vi "create_process_list (SubVI).vi"(0 "Synth settings:":T1={"start volt (V)"=1.0, "stop volt (V) "=1.0, "# V Steps"=1, "start freq (Hz)"=2000.0, "stop freq (Hz) "=2000.0, "# F steps"=1, "dc offset?"=FALSE, "start DC (V)"=0.5, "stop DC (V)"=0.5, "# DC steps "=1, "Set synth\n(HP33120A)?"=FALSE, "Use arbitrary\nwaveform?"=FALSE, "Arb waveform name:"=""}, 1 "DC supply settings:":T5, 2 "Electrode settings:":T2={"DC volts (V):\n"=[], "Electrode to sweep:"=0, "start volt (V)"=0.0, "stop volt (V) "=0.0, "# V Steps"=1, "start freq (Hz)"=41.0, "stop freq (Hz) "=41.0, "# F steps"=1, "start DC (V)"=0.0, "stop DC (V)"=0.0, "# DC steps "=1, "Digitize electrode\ndrives?"=FALSE, "Sweep electrode?"=FALSE, "Add 0.5*V DC \noffset for amp?"=FALSE, "Use electrode \nconfig file?"=FALSE, "Path"=path ""}, 3 "Stage settings:":T3={"Set stage?"=FALSE, "start X (um)"=0.0, "stop X (um) "=0.0, "# X Steps"=1, "start Y (um)"=0.0, "stop Y (um) "=0.0, "# Y steps"=1, "start Z (um)"=0.0, "stop Z (um)"=0.0, "# Z steps "=1, "Sweep?"=FALSE, "Dir to sweep"=0, "Amplitude (um)"=0.0, "Frequency (Hz)"=41.0} {"Dir to sweep" items=["X", "Y", "Z"]}) -> (6 "Process list":T4(array[cluster]))   [LabVIEW 2014]
panel:
  # "0"
  # "1"
  # "2"
  # "3"
  # "4"
  # "5"
  # "6"
  # "7"
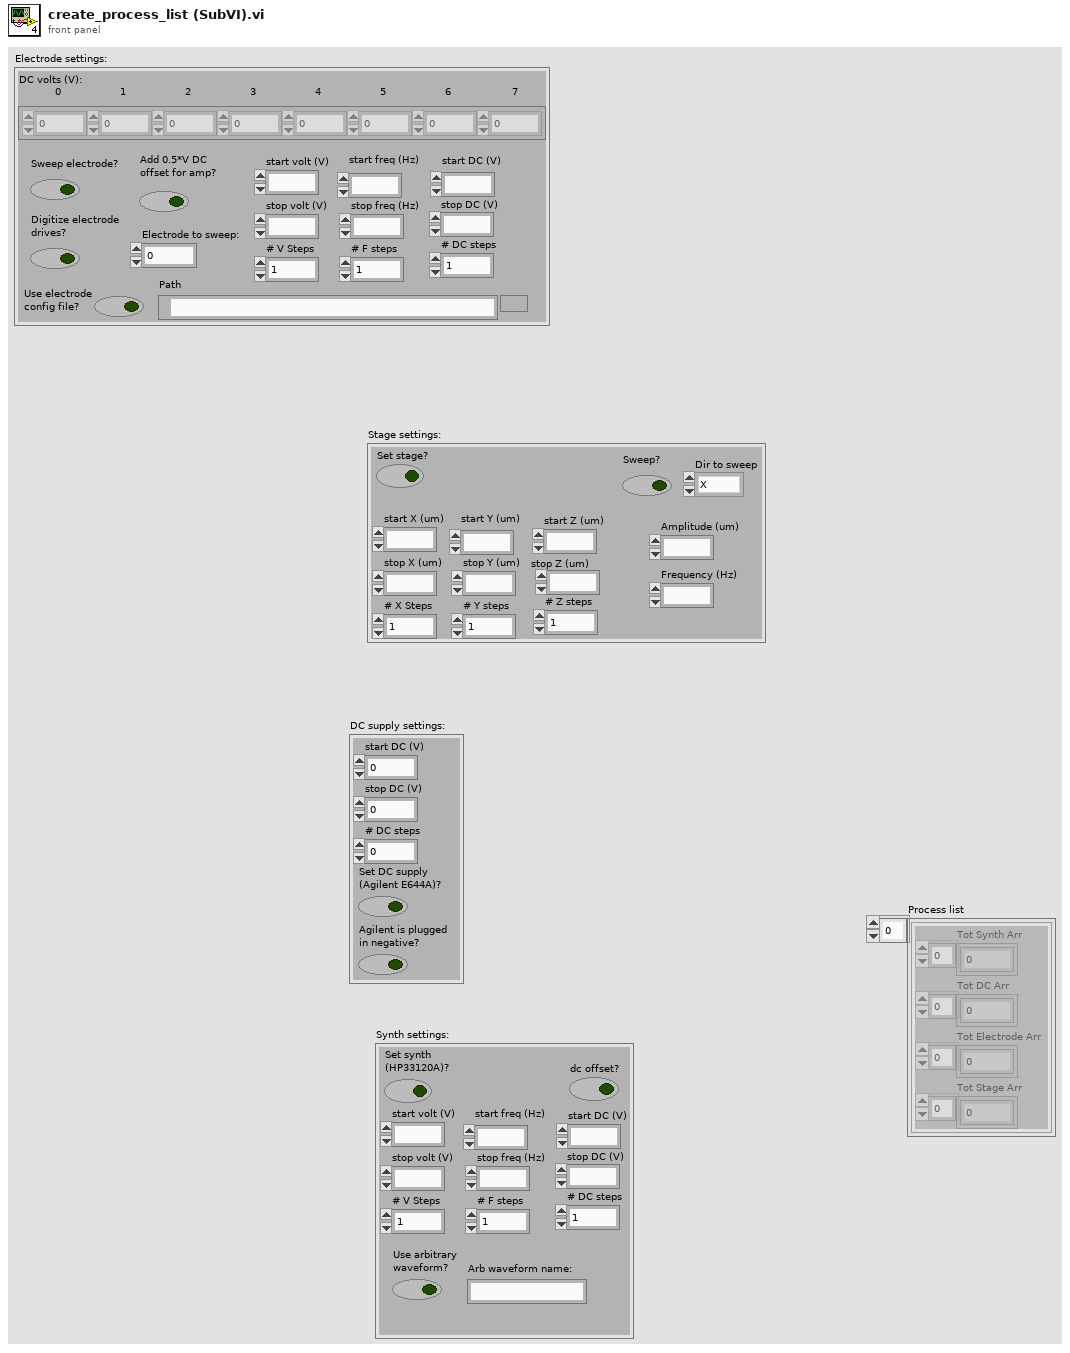
[diagram p1: front panel]
types:
  T1 = cluster{"start volt (V)":ext, "stop volt (V) ":ext, "# V Steps":i32, "start freq (Hz)":ext, "stop freq (Hz) ":ext, "# F steps":i32, "dc offset?":bool, "start DC (V)":ext, "stop DC (V)":ext, "# DC steps ":i32, "Set synth\n(HP33120A)?":bool, "Use arbitrary\nwaveform?":bool, "Arb waveform name:":string}
  T2 = cluster{"DC volts (V):\n":dbl[], "Electrode to sweep:":i32, "start volt (V)":ext, "stop volt (V) ":ext, "# V Steps":i32, "start freq (Hz)":ext, "stop freq (Hz) ":ext, "# F steps":i32, "start DC (V)":ext, "stop DC (V)":ext, "# DC steps ":i32, "Digitize electrode\ndrives?":bool, "Sweep electrode?":bool, "Add 0.5*V DC \noffset for amp?":bool, "Use electrode \nconfig file?":bool, "Path":path}
  T3 = cluster{"Set stage?":bool, "start X (um)":ext, "stop X (um) ":ext, "# X Steps":i32, "start Y (um)":ext, "stop Y (um) ":ext, "# Y steps":i32, "start Z (um)":ext, "stop Z (um)":ext, "# Z steps ":i32, "Sweep?":bool, "Dir to sweep":u16, "Amplitude (um)":ext, "Frequency (Hz)":ext}
  T4 = cluster{"Tot Synth Arr":dbl[], "Tot DC Arr":dbl[], "Tot Electrode Arr":dbl[], "Tot Stage Arr":dbl[]}[]
  T5 = cluster{"start DC (V)":ext, "stop DC (V)":ext, "# DC steps ":i32, "Set DC supply\n(Agilent E644A)? ":bool, "Agilent is plugged \nin negative?":bool}
  T6 = cluster{"Tot Synth Arr":dbl[], "Tot DC Arr":dbl[], "Tot Electrode Arr":dbl[], "Tot Stage Arr":dbl[]}
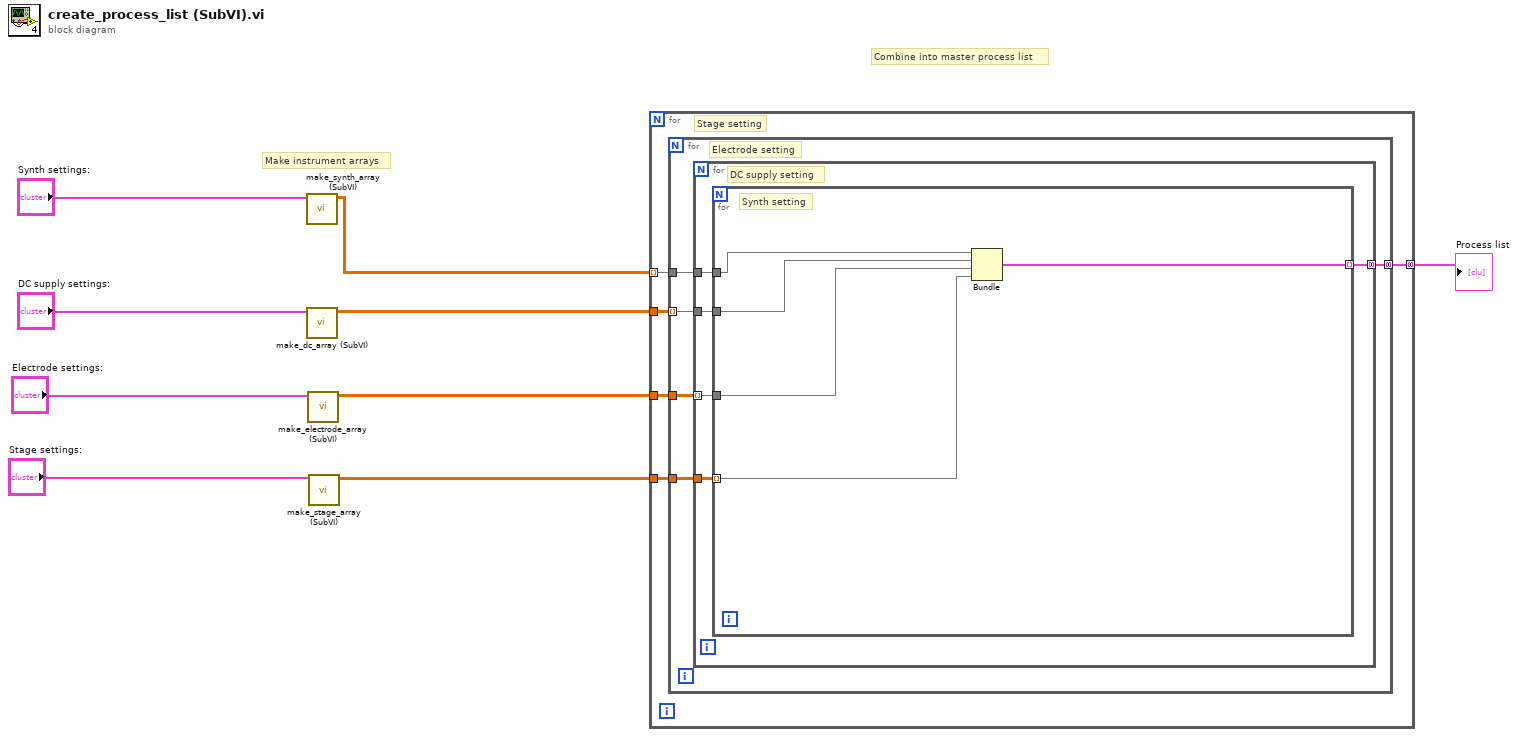
[diagram p0: block diagram]
diagram:
  # "Combine into master process list"
  # "Make instrument arrays"
  n1 = call "make_synth_array (SubVI).vi"("Synth settings:"="Synth settings:") -> ("Tot Synth Arr"=w8:dbl[][])  [unwired: 10 in]
  n2 = call "make_dc_array (SubVI).vi"("DC supply settings:"="DC supply settings:") -> ("Tot DC Arr"=w7:dbl[][])  [unwired: 10 in]
  n3 = call "make_electrode_array (SubVI).vi"("Electrode settings:"="Electrode settings:") -> ("Tot Electrode Arr"=w6:dbl[][])  [unwired: 10 in]
  n4 = call "make_stage_array (SubVI).vi"("Stage settings:"="Stage settings:") -> ("Tot Stage Arr"=w5:dbl[][])  [unwired: 10 in]
  n5 = for {
    tunnel: w8 -> [w14] mode=indexing
    tunnel: w7 -> [w13]
    tunnel: w6 -> [w12]
    tunnel: w5 -> [w11]
    tunnel: [w10] -> w4 mode=concatenating
    # "Stage setting"
    n6 = for {
      tunnel: w14 -> [w19]
      tunnel: w13 -> [w18] mode=indexing
      tunnel: w12 -> [w17]
      tunnel: w11 -> [w16]
      tunnel: [w15] -> w10 mode=concatenating
      # "Electrode setting"
      n7 = for {
        tunnel: w19 -> [w24]
        tunnel: w18 -> [w23]
        tunnel: w17 -> [w22] mode=indexing
        tunnel: w16 -> [w21]
        tunnel: [w20] -> w15 mode=concatenating
        # "DC supply setting"
        n8 = for {
          tunnel: w24 -> [w25]
          tunnel: w23 -> [w29]
          tunnel: w22 -> [w28]
          tunnel: w21 -> [w27] mode=indexing
          tunnel: [w26] -> w20 mode=indexing
          # "Synth setting"
          n9 = Bundle("Tot Synth Arr"=w25, "Tot DC Arr"=w29, "Tot Electrode Arr"=w28, "Tot Stage Arr"=w27) -> (w26:T6)  [unwired: 1 in]
        }
      }
    }
  }
  "Process list" <- w4
